vi "test Pulse Width Modulation.vi"(8 "error in (no error)":errorcluster, 11 "TestCase in":refnum<class "Scan Engine Specialty Digital System Tests.lvclass">) -> (0 "error out":errorcluster, 3 "TestCase out":refnum<class "Scan Engine Specialty Digital System Tests.lvclass">)   [LabVIEW 2019, in "Scan Engine Specialty Digital System Tests.lvclass"]
uses:
  Scan Engine Specialty Digital System Tests.lvclass
  C:/Users/nitest/Desktop/Git 2019/niveristand-custom-device-testing-tools/VeriStandTestCase/VeriStandTestCase.lvclass
  <vilib>/addons/_JKI Toolkits/VI Tester/TestCase.llb/TestCase.lvclass
  niveristand-custom-device-testing-tools/VeriStandTestUtilities/VeriStandTestUtilities.lvlib
  C:/Program Files (x86)/National Instruments/LabVIEW 2019/vi.lib/addons/_JKI Toolkits/VI Tester/TestCase.llb/TestCase.lvclass
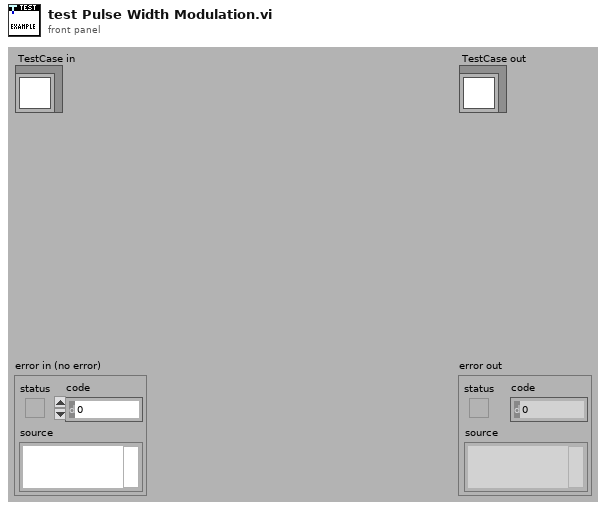
[diagram p1: front panel]
types:
  T1 = typedef "NI_VS Workspace ExecutionAPI.lvlib/WorkspaceAPI.ctl" = refnum<k24>
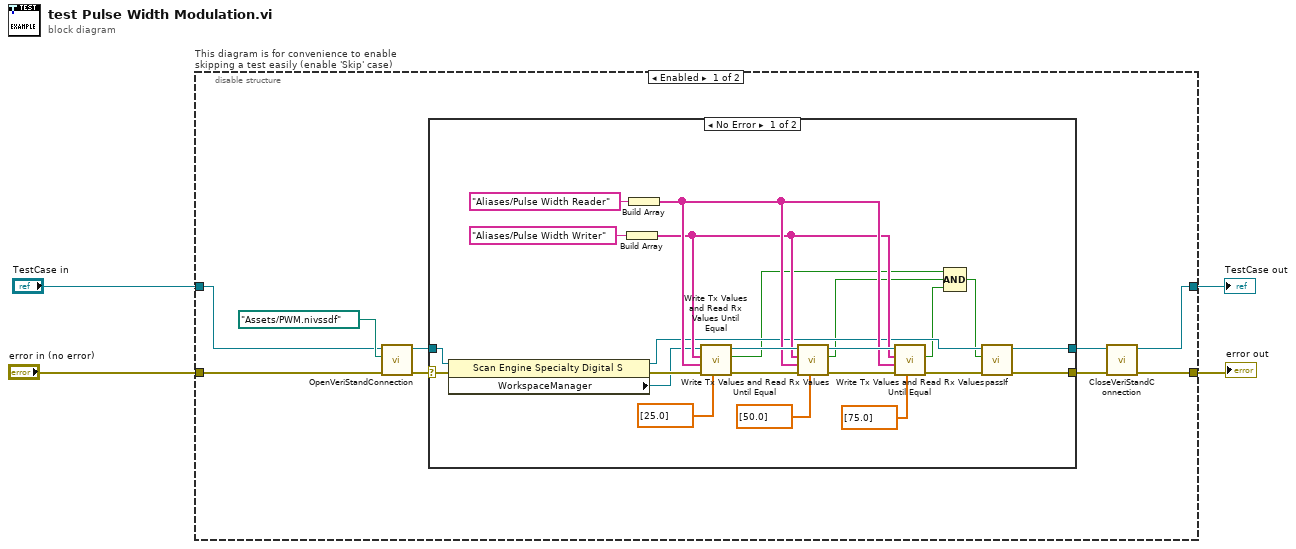
[diagram p0: block diagram]
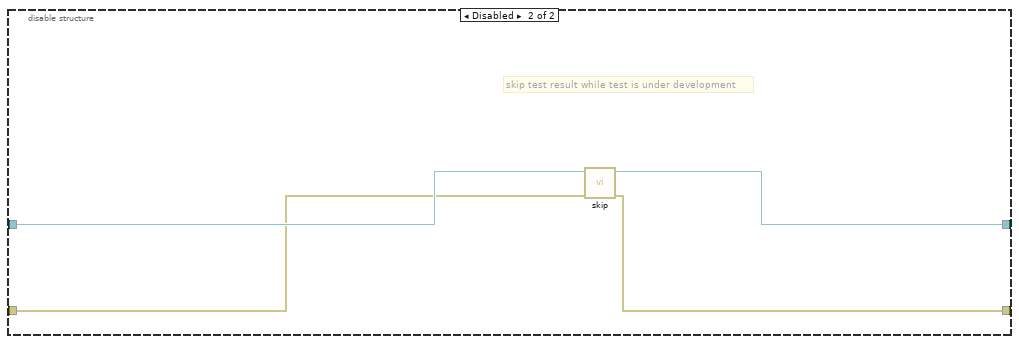
[diagram p3: hidden frame]
diagram:
  n1 = disable-structure "This diagram is for convenience to enable skipping a test easily (enable 'Skip' case)" shown="Enabled" {
    disable-tunnel: "TestCase in" -> [w9 w42]
    disable-tunnel: [w6 w40] -> w1
    disable-tunnel: [w7 w41] -> w3
    disable-tunnel: "error in (no error)" -> [w11 w39]
    frame Enabled {
      n2 = call-dynamic "OpenVeriStandConnection.vi"("error in (no error)"=w11, "System Definition File"=path "Assets/PWM.nivssdf", "VeriStand Test Case in"=w9) -> ("error out"=w12:errorcluster, "VeriStand Test Case out"=w10:refnum<class "Scan Engine Specialty Digital System Tests.lvclass">)  [unwired: 6 in, 1 out]
      n3 = case shown="No Error" w12 {
        selector: w12 -> [w26 w38]
        tunnel: [w20 w38] -> w8
        tunnel: w10 -> [w27 w37]
        tunnel: [w18 w37] -> w5
        frame No Error {
          n4 = property class="Scan Engine Specialty Digital S"(reference=w27, error in=w26) -> (reference out=w19:refnum<class "Scan Engine Specialty Digital System Tests.lvclass">, error out=w25:errorcluster, "WorkspaceManager"=w24:T1)
          n5 = Build Array("Aliases/Pulse Width Writer" ("Channel")) -> (w28:string[])
          n6 = Build Array("Aliases/Pulse Width Reader" ("Channel")) -> (w29:string[])
          n7 = call "Write Tx Values and Read Rx Values Until Equal.vi"("Tx values"=dbl[] [25.0], "error in"=w25, "Rx aliases"=w29, "Tx aliases"=w28, "workspace manager in"=w24) -> ("error out"=w35:errorcluster, "values equal"=w17:bool, "workspace manager out"=w36:T1)  [unwired: 4 in]
          n8 = call "Write Tx Values and Read Rx Values Until Equal.vi"("Tx values"=dbl[] [50.0], "error in"=w35, "Rx aliases"=w29, "Tx aliases"=w28, "workspace manager in"=w36) -> ("error out"=w33:errorcluster, "values equal"=w16:bool, "workspace manager out"=w34:T1)  [unwired: 4 in]
          n9 = call "Write Tx Values and Read Rx Values Until Equal.vi"("Tx values"=dbl[] [75.0], "error in"=w33, "Rx aliases"=w29, "Tx aliases"=w28, "workspace manager in"=w34) -> ("error out"=w32:errorcluster, "values equal"=w15:bool)  [unwired: 4 in, 1 out]
          n10 = Compound Arithmetic op=AND(w17, w16, w15) -> (w14:bool)
          n11 = call-dynamic "passIf.vi"("error in (no error)"=w32, "pass"=w14, "TestCase in"=w19) -> ("error out"=w20:errorcluster, "TestCase out"=w18:refnum<class "Scan Engine Specialty Digital System Tests.lvclass">)  [unwired: 7 in]
        }
        frame Error {
        }
      }
      n12 = call-dynamic "CloseVeriStandConnection.vi"("error in (no error)"=w8, "VeriStand Test Case in"=w5) -> ("error out"=w7:errorcluster, "VeriStand Test Case out"=w6:refnum<class "Scan Engine Specialty Digital System Tests.lvclass">)  [unwired: 8 in]
    }
    frame Disabled {
      # "skip test result while test is under development"
      n13 = call <vilib>:"skip.vi"("error in (no error)"=w39, "TestCase in"=w42) -> ("error out"=w41:errorcluster, "TestCase out"=w40:refnum<class "Scan Engine Specialty Digital System Tests.lvclass">)  [unwired: 8 in]
    }
  }
  "error out" <- w3
  "TestCase out" <- w1
